vi "ATS_NumOfSystem.vi"() -> (3 "Num_Of_System":u32)   [LabVIEW 2014]
doc: "_____AlazarTech, Scope_____\n\nReturn the total number of Master/Slave and independent board system."
uses:
  ATSApi.dll
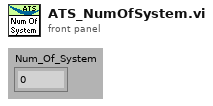
[diagram p1: front panel]
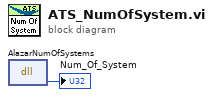
[diagram p0: block diagram]
diagram:
  n1 = dll-call lib="D:/IntensityOCT/trunk/ATSApi.dll" fn="AlazarNumOfSystems"() -> (→"Num_Of_System":u32)  [unwired: 3 in, 2 out]
